vi "Set Default VI Icon Properties.vi"(8 "error in (no error)":errorcluster, 10 "Save VI (T)":bool=TRUE, 11 "vi path":path) -> (0 "error out":errorcluster)   [LabVIEW 2023]
uses:
  <vilib>/LabVIEW Icon API/lv_icon/Controls/BodyText.ctl
  <vilib>/LabVIEW Icon API/lv_icon/Controls/Font.ctl
  <vilib>/LabVIEW Icon API/lv_icon/Controls/Alignment.ctl
  <vilib>/LabVIEW Icon API/LabVIEW Icon API.lvlib
  <vilib>/LabVIEW Icon API/lv_icon/lv_icon.lvlib
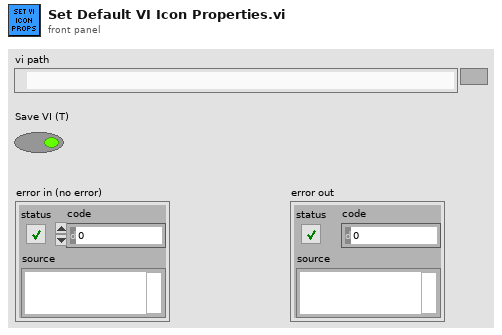
[diagram p1: front panel]
types:
  T1 = typedef "Alignment.ctl" = u16
  T2 = typedef "Font.ctl" = string
  T3 = typedef "BodyText.ctl" = cluster{"Line 1 text":string, "Line 2 text":string, "Line 3 text":string, "Line 4 text":string, "Line 1 color":u32, "Line 2 color":u32, "Line 3 color":u32, "Line 4 color":u32, "Body Text Spec":cluster{"Font":T2, "Alignment":T1, "Size":u8}, "Center text vertically":bool, "Capitalize Text":bool}
  T4 = typedef "LabVIEW Icon Stored Information.ctl" = cluster{"Text Visible?":bool, "Text Opacity":u8, "Templ Visible?":bool, "Templ Opacity":u8, "Relative Path from 1 to 2":path, "Image":picture, "All User Layers":refnum<class "Layer.lvclass">[], "Body Text":T3}
  T5 = typedef "imagedata.ctl" = cluster{"image type":i32, "image depth":i32, "image":u8[], "mask":u8[], "colors":u32[], "Rectangle":cluster{"left":i16, "top":i16, "right":i16, "bottom":i16}}
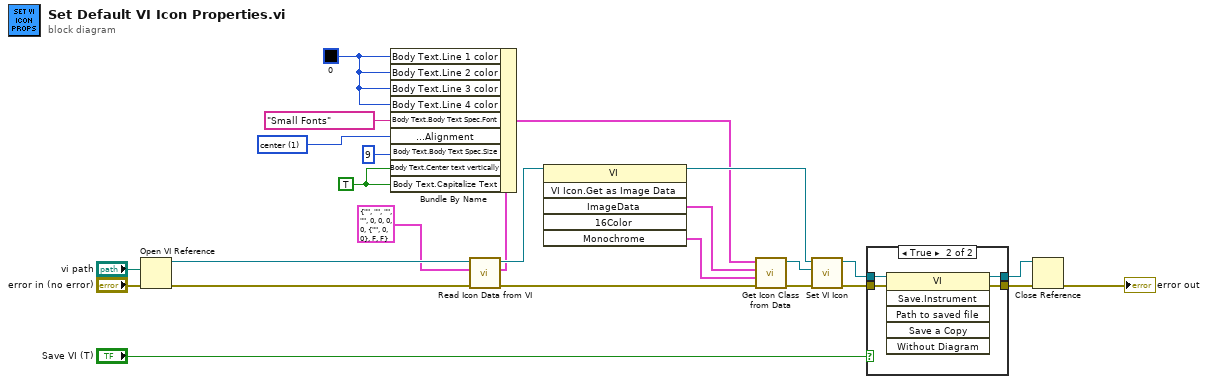
[diagram p0: block diagram]
diagram:
  w7 = T1 1 items=["left", "center", "right"] ("Body Text.Body Text Spec.Alignment")
  w9 = TRUE ("Body Text.Center text vertically")
  w10 = u32 0
  n1 = Open VI Reference(vi path="vi path", error in (no error)="error in (no error)") -> (vi reference=w25:refnum<vi>, error out=w4:errorcluster)  [unwired: 4 in]
  n2 = call <vilib>:"Read Icon Data from VI.vi"("error in (no error)"=w4, "Default body text"=T3 {"Line 1 text"="", "Line 2 text"="", "Line 3 text"="", "Line 4 text"="", "Line 1 color"=0, "Line 2 color"=0, "Line 3 color"=0, "Line 4 color"=0, "Body Text Spec"={"Font"="", "Alignment"=0, "Size"=0}, "Center text vertically"=FALSE, "Capitalize Text"=FALSE}, "VI Ref in"=w25) -> ("error out"=w24:errorcluster, "Data"=w14:T4, "VI Ref out"=w17:refnum<vi>)  [unwired: 6 in]
  n3 = Bundle By Name(cluster=w14, "Body Text.Line 1 color"=w10, "Body Text.Line 2 color"=w10, "Body Text.Line 3 color"=w10, "Body Text.Line 4 color"=w10, "Body Text.Body Text Spec.Font"=T2 "Small Fonts", "Body Text.Body Text Spec.Alignment"=w7, "Body Text.Body Text Spec.Size"=u8 9, "Body Text.Center text vertically"=w9, "Body Text.Capitalize Text"=w9) -> (w5:T4)
  n4 = invoke class="VI" method="VI Icon.Get as Image Data"(reference=w17) -> (reference out=w12:refnum<vi>, "ImageData"=w16:T5, "Monochrome"=w15:T5)  [unwired: 5 in, 3 out]
  n5 = call <vilib>:"Get Icon Class from Data.vi"("error in (no error)"=w24, "BW Icon"=w15, "Color Icon"=w16, "Icon Data"=w5) -> ("error out"=w11:errorcluster, "Icon out"=w13:refnum<class "Icon.lvclass">)  [unwired: 6 in]
  n6 = call <vilib>:"Set VI Icon.vi"("error in (no error)"=w11, "Icon"=w13, "VI Refnum in"=w12) -> ("error out"=w2:errorcluster, "VI Refnum out"=w1:refnum<vi>)  [unwired: 7 in]
  n7 = case shown="True" "Save VI (T)" {
    tunnel: [w26 w28] -> w21
    tunnel: [w27 w31] -> w20
    tunnel: w2 -> [w26 w29]
    tunnel: w1 -> [w27 w30]
    frame False {
    }
    frame True {
      n8 = invoke class="VI" method="Save.Instrument"(reference=w30, error in=w29) -> (reference out=w31:refnum<vi>, error out=w28:errorcluster)  [unwired: 4 in, 4 out]
    }
  }
  n9 = Close Reference(reference=w20, error in (no error)=w21) -> (error out=→"error out":errorcluster)
